vi "Write Boolean.vi"(8 "error in":errorcluster, 9 "value in":bool, 10 "register offset":u32, 11 "session in":u32) -> (0 "error out":errorcluster, 3 "session out":u32)   [LabVIEW 2018, in "Scalar IO Operations.lvlib"]
uses:
  Scalar IO Operations.lvlib
  NiFpga.dll
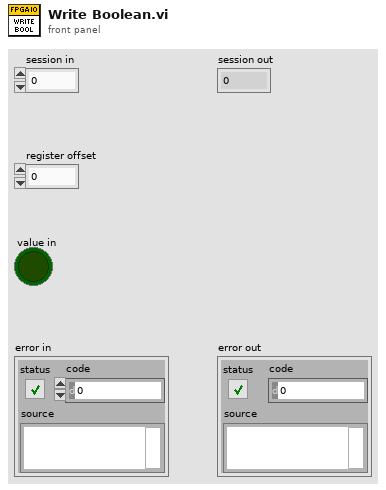
[diagram p1: front panel]
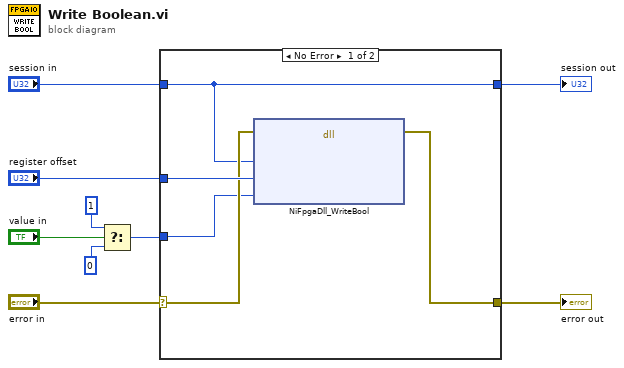
[diagram p0: block diagram]
diagram:
  n1 = Select(t=u8 1 ("value"), s="value in", f=u8 0) -> (s? t:f=w1:u8)
  n2 = case shown="No Error" "error in" {
    selector: "error in" -> [w12 w16]
    tunnel: "session in" -> [w11 w15]
    tunnel: [w14 w16] -> w8
    tunnel: "register offset" -> [w13 _]
    tunnel: [w11 w15] -> w5
    tunnel: w1 -> [w10 _]
    frame No Error {
      n3 = dll-call lib="NiFpga.*" fn="NiFpgaDll_WriteBool"(error in=w12, "session"=w11, "offset"=w13, "value"=w10) -> (error out=w14:errorcluster)  [unwired: 6 in, 1 out]
    }
    frame Error {
    }
  }
  "error out" <- w8
  "session out" <- w5
